vi "PH_DIM.Event Declarer.vi"(1 "Selector":string, 2 "Service Name":string) -> (0 "declared DIM Event":T1)   [LabVIEW 2014, in "PH_Common.lvlib"]
doc: "This VI is nothing but a short cut of a bit of code often used in ProcEvents."
uses:
  PH_Common.lvlib
  PH_DIM.Event Declarer.ctl
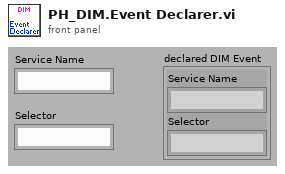
[diagram p1: front panel]
types:
  T1 = typedef "PH_Common.lvlib/PH_DIM.Event Declarer.ctl" = cluster{"Service Name":string, "Selector":string}
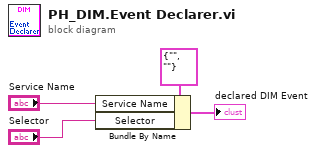
[diagram p0: block diagram]
diagram:
  n1 = Bundle By Name(cluster=T1 {"Service Name"="", "Selector"=""} ("DIM Event Declarer"), "Service Name"="Service Name", "Selector"="Selector") -> (→"declared DIM Event":T1)
